vi "Make Rotation Matrix.vi"(10 "Rotation Axis":dbl[](array[numeric])=[1.0, 0.0, 0.0], 11 "Rotation Angle (Degree)":dbl=90.0) -> (3 "Rotation Matrix":T1=[[1.0, 0.0, 0.0], [0.0, 6.123233995736766e-17, 1.0], [0.0, -1.0, 6.123233995736766e-17]])   [LabVIEW 2010]
uses:
  <vilib>/Analysis/Matrix/Datatypes/RealMatrix.ctl
  <vilib>/Analysis/Matrix/Numeric/Multiply/Multiply - R,RM.vi
  <vilib>/Analysis/baseanly.llb/Real Outer Product.vi
  <vilib>/Analysis/Matrix/Numeric/Add/Add - RM,RM.vi
  <vilib>/Analysis/NI_AALBase.lvlib
  <vilib>/Analysis/Matrix/NI_Matrix.lvlib
panel:
  out "Cross Product Matrix":T1=[[0.0, 0.0, -0.0], [-0.0, 0.0, 1.0], [0.0, -1.0, 0.0]]
  out "Outer Product":T1=[[1.0, 0.0, 0.0], [0.0, 0.0, 0.0], [0.0, 0.0, 0.0]]
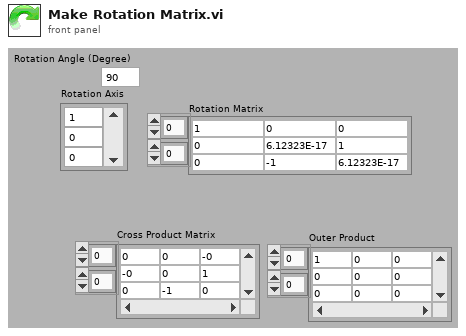
[diagram p1: front panel]
types:
  T1 = typedef "NI_Matrix.lvlib/RealMatrix.ctl" = dbl[][]
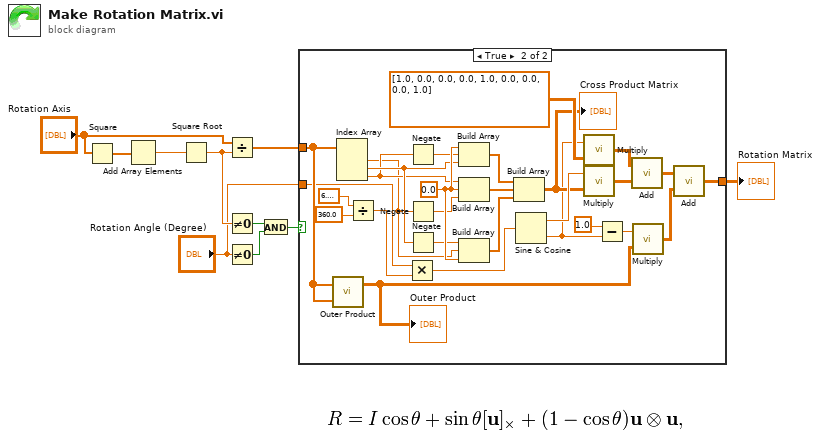
[diagram p0: block diagram]
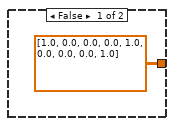
[diagram p2: hidden frame]
diagram:
  n1 = Square(x="Rotation Axis") -> (x^2=w7:dbl[])
  n2 = Add Array Elements(numeric array=w7) -> (sum=w8:dbl)
  n3 = Square Root(x=w8) -> (sqrt(x)=w5:dbl)
  n4 = Divide(x="Rotation Axis", y=w5) -> (x/y=w10:dbl[])
  n5 = Not Equal To 0?(x=w5) -> (x != 0?=w3:bool)
  n6 = Not Equal To 0?(x="Rotation Angle (Degree)") -> (x != 0?=w2:bool)
  n7 = And(x=w3, y=w2) -> (x .and. y?=w1:bool)
  n8 = case shown="True" w1 {
    tunnel: w10 -> [_ w34]
    tunnel: [T1 [[1.0, 0.0, 0.0], [0.0, 1.0, 0.0], [0.0, 0.0, 1.0]] ("A + B") w13] -> w9
    tunnel: "Rotation Angle (Degree)" -> [_ w12]
    frame False {
    }
    frame True {
      w33 = 0.0 ("element")
      n9 = call-poly <vilib>:"Outer Product.vi"("Y Vector"=w34, "X Vector"=w34) -> ("Outer Product"=w15:T1)  [unwired: 1 out]
      "Outer Product" <- w15
      n10 = Index Array(array=w34) -> (element #1=w25:dbl, element #2=w29:dbl, element #3=w28:dbl)  [unwired: 3 in]
      n11 = Divide(x=6.283185307179586, y=360.0) -> (x/y=w38:dbl)
      n12 = Multiply(x=w12, y=w38) -> (x*y=w39:dbl)
      n13 = Negate(x=w28) -> (-x=w30:dbl)
      n14 = Negate(x=w25) -> (-x=w27:dbl)
      n15 = Negate(x=w29) -> (-x=w26:dbl)
      n16 = Build Array(w33, w30, w29) -> (w35:dbl[])
      n17 = Build Array(w28, w33, w27) -> (w32:dbl[])
      n18 = Build Array(w26, w25, w33) -> (w31:dbl[])
      n19 = Build Array(w35, w32, w31) -> (w21:T1)
      "Cross Product Matrix" <- w21
      n20 = Sine & Cosine(0:w39) -> (1:w22:dbl, 2:w17:dbl)
      n21 = call-poly <vilib>:"Multiply.vi"("Real Matrix A"=T1 [[1.0, 0.0, 0.0], [0.0, 1.0, 0.0], [0.0, 0.0, 1.0]] ("X Rotation Matrix 2"), "Real Scalar c"=w17) -> ("c * A"=w23:T1)
      n22 = call-poly <vilib>:"Multiply.vi"("Real Matrix A"=w21, "Real Scalar c"=w22) -> ("c * A"=w20:T1)
      n23 = Subtract(x=1.0, y=w17) -> (x-y=w16:dbl)
      n24 = call-poly <vilib>:"Add.vi"("Real Matrix B"=w20, "Real Matrix A"=w23) -> ("A + B"=w19:T1)
      n25 = call-poly <vilib>:"Multiply.vi"("Real Matrix A"=w15, "Real Scalar c"=w16) -> ("c * A"=w14:T1)
      n26 = call-poly <vilib>:"Add.vi"("Real Matrix B"=w14, "Real Matrix A"=w19) -> ("A + B"=w13:T1)
    }
  }
  "Rotation Matrix" <- w9
